vi "Parse Core(override).vi"(8 "error in (no error)":errorcluster, 11 "TXT in":refnum<class "TXT.lvclass">=refnum) -> (0 "error out":errorcluster, 2 "Dictionaries Out":refnum<class "String Database.lvclass">[](array[class]), 3 "TXT out":refnum<class "TXT.lvclass">)   [LabVIEW 2016, in "TXT.lvclass"]
uses:
  TXT.lvclass
  Includes/String Database/String Database.lvlibp/String Database.lvclass
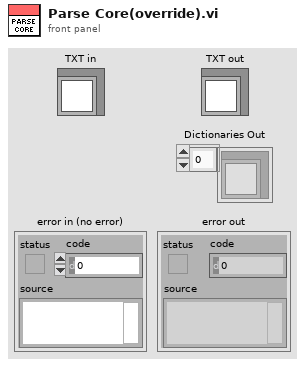
[diagram p1: front panel]
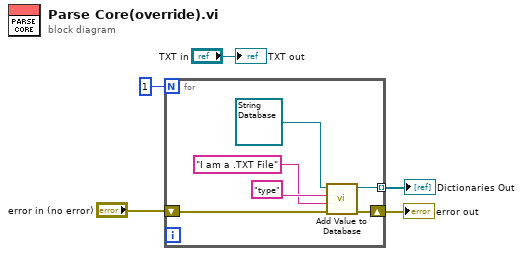
[diagram p0: block diagram]
diagram:
  n1 = for {
    N: 1 -> [_]
    tunnel: [w9] -> w2 mode=indexing
    shift-right: [w10] -> w3
    shift-left: "error in (no error)" -> [w11]
    n2 = call "Add Value to Database.vi"("error in (no error)"=w11, "Entry Value"="I am a .TXT File", "Entry Name"="type", "Dictionary In"=refnum<class "String Database.lvclass"> refnum ("Message in")) -> ("error out"=w10:errorcluster, "Dictionary Out"=w9:refnum<class "String Database.lvclass">)  [unwired: 5 in, 1 out]
  }
  "error out" <- w3
  "Dictionaries Out" <- w2
  "TXT out" <- "TXT in"
